vi "Channel Measurement Limit Add.vi"(4 "EndYVal":dbl, 5 "BeginYVal":dbl, 6 "EndXVal":dbl, 7 "BeginXVal":dbl, 8 "error in (no error)":errorcluster {"code" format="%.0x"}, 9 "LimitTypeVal (Off)":i32(ring) items=["Off", "Maximum", "Minimum"], 10 "RepCapIdentifier":string, 11 "instrument handle":refnum<k15>) -> (0 "error out":errorcluster {"code" format="%.0x"}, 3 "instrument handle out":refnum<k15>)   [LabVIEW 2014, in "Agilent NA.lvlib"]
doc: "Inserts or appends a new limit line in the limit table at the position specified by the Number property. If Number is greater than the number of limits currently defined, Number is set to the next available position in the limit table."
uses:
  Agilent NA.lvlib
  AgNA.dll
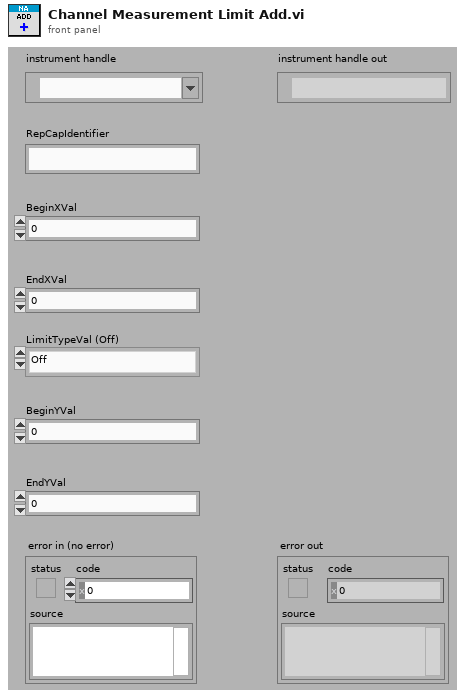
[diagram p1: front panel]
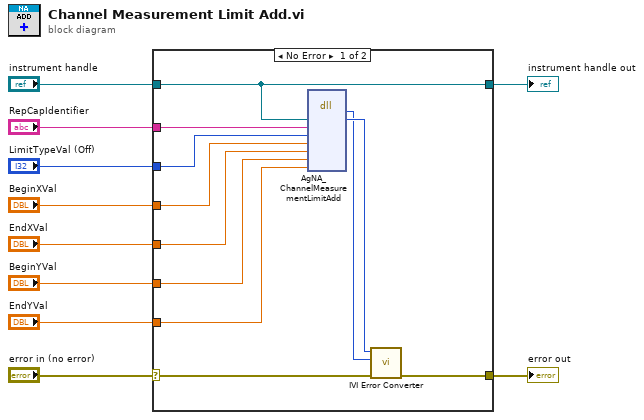
[diagram p0: block diagram]
diagram:
  n1 = case shown="No Error" "error in (no error)" {
    selector: "error in (no error)" -> [w19 w23]
    tunnel: [w18 w23] -> w10
    tunnel: "RepCapIdentifier" -> [w17 _]
    tunnel: "LimitTypeVal (Off)" -> [w16 _]
    tunnel: "BeginXVal" -> [w15 _]
    tunnel: "EndXVal" -> [w14 _]
    tunnel: "BeginYVal" -> [w13 _]
    tunnel: "EndYVal" -> [w12 _]
    tunnel: [w11 w22] -> w1
    tunnel: "instrument handle" -> [w11 w22]
    frame No Error {
      n2 = dll-call lib="AgNA**.dll" fn="AgNA_ChannelMeasurementLimitAdd"("Vi"=w11, "RepCapIdentifier"=w17, "LimitTypeVal"=w16, "BeginXVal"=w15, "EndXVal"=w14, "BeginYVal"=w13, "EndYVal"=w12) -> (w20:i32, "Vi"=w21:u32)  [unwired: 9 in, 2 out]
      n3 = call "IVI Error Converter.vi"("error in (no error)"=w19, "IVI error code (0)"=w20, "instrument handle"=w21) -> ("error out"=w18:errorcluster)  [unwired: 7 in, 1 out]
    }
    frame Error {
    }
  }
  "error out" <- w10
  "instrument handle out" <- w1
